vi "Dialog Box.vi"(8 "error in (no error)":errorcluster, 11 "Serial Number":string) -> (0 "error out":errorcluster)   [LabVIEW 2015]
panel:
  out "Serial Number 2":string
  in  "OK Button":bool
  out "Test Sequence":i32(listbox)=-2
  # "OC User Action Needed"
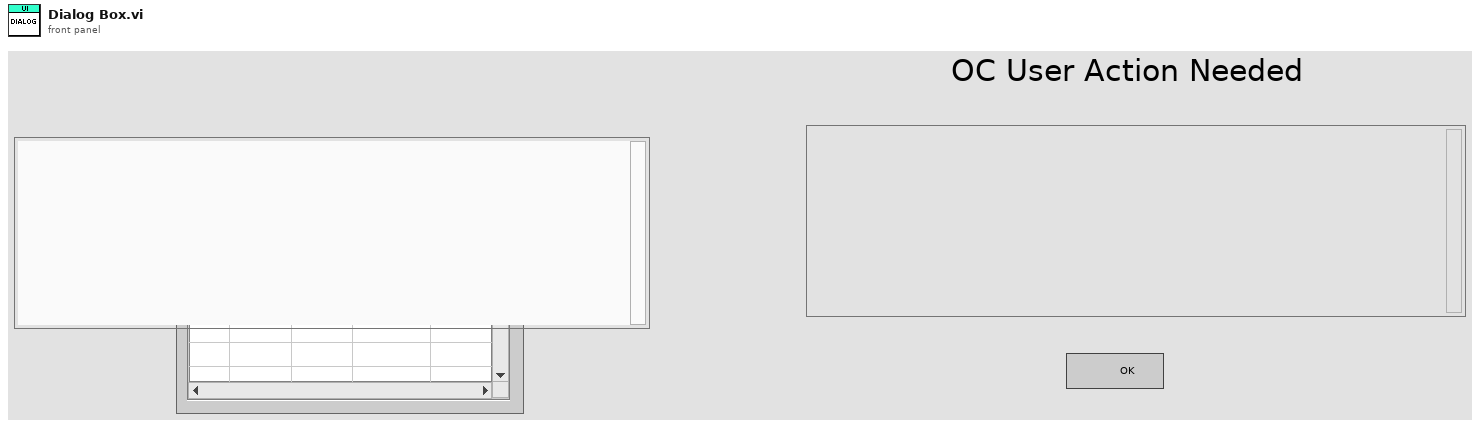
[diagram p1: front panel]
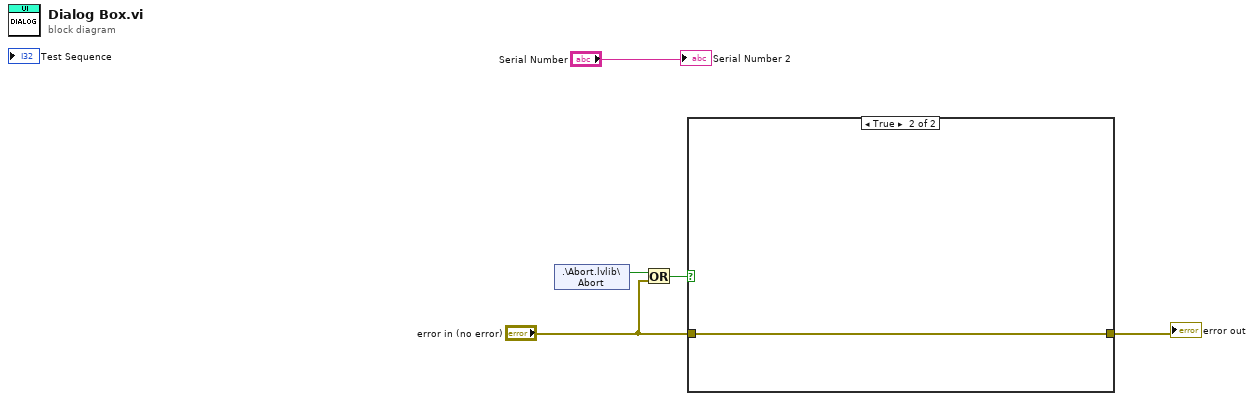
[diagram p0: block diagram]
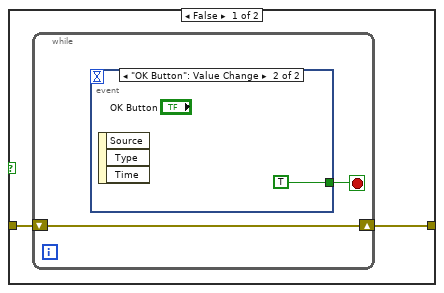
[diagram p2: hidden frame]
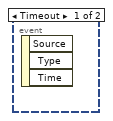
[diagram p3: hidden frame]
diagram:
  n1 = shared-variable ".\\Abort.lvlib\\Abort"() -> (w4:bool)  [unwired: 1 in, 1 out]
  n2 = Or(x=w4, y="error in (no error)") -> (x .or. y?=w3:bool)
  n3 = case shown="True" w3 {
    tunnel: [w7 w11] -> w5
    tunnel: "error in (no error)" -> [w6 w11]
    frame False {
      n4 = while {
        shift-right: [w8] -> w7
        shift-left: w6 -> [w8]
        stop <- w9 stop-if-true
        n5 = event shown="[1] \"OK Button\": Value Change" {
          selector: _ -> [_ _]
          dyn-events: _ -> [_ _]
          timeout: _ -> [_ _]
          tunnel: [_ TRUE] -> w9
          event Timeout {
            n6 = event-data() -> ()  [unwired: 1 in, 3 out]
          }
          event "OK Button": Value Change {
            n7 = event-data() -> ()  [unwired: 1 in, 3 out]
          }
        }
      }
    }
    frame True {
    }
  }
  "error out" <- w5
  "Serial Number 2" <- "Serial Number"
